vi "Test Class String IDs.vi"() -> ()   [LabVIEW 2018, in "Test.lvclass"]
uses:
  Test.lvclass
panel:
  in  "Tab Control":enum32{"General", "Config ID's"}(tab)
  in  "Comparison Value Constant Name":string="Comparison Value"
  in  "Sequence ID":string="Sequence"
  in  "Additional Data Constant Name":string="Additional Data"
  in  "Comparison Value 2":string="CompVal_2"
  in  "Comparison Value 1":string="CompVal_1"
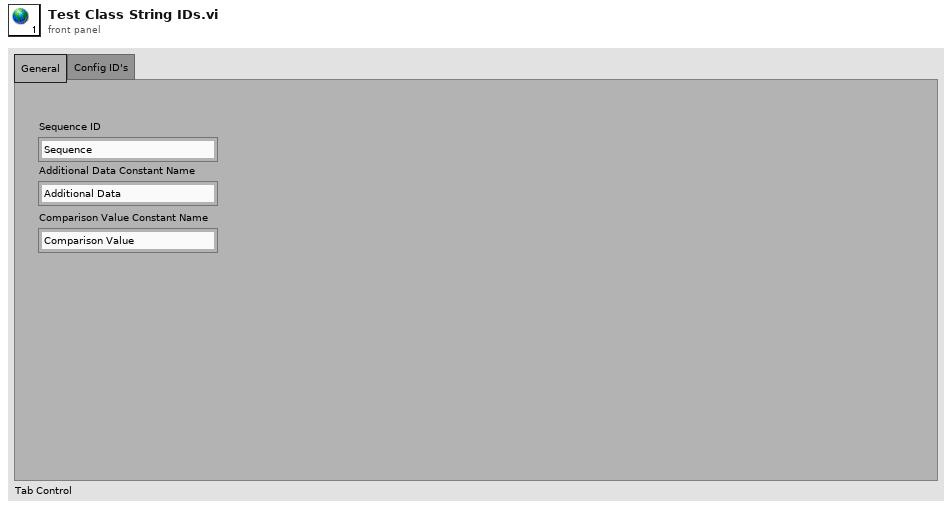
[diagram p1: front panel]
diagram:
